vi "Create Folder.vi"(0 "Directory Path":path, 11 "error in (no error)":errorcluster) -> (4 "Dup Directory Path":path, 15 "error out":errorcluster)   [LabVIEW 2021, in "Path Functions.lvlib"]
uses:
  Path Functions.lvlib
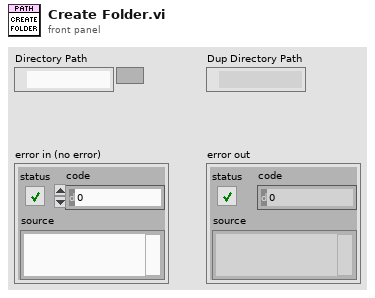
[diagram p1: front panel]
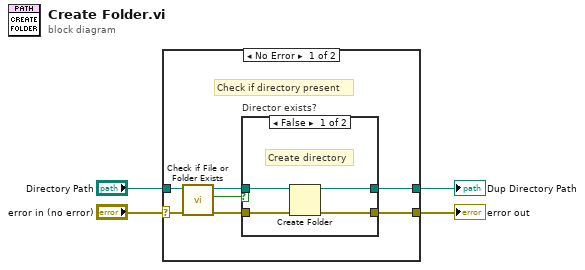
[diagram p0: block diagram]
diagram:
  n1 = case shown="No Error" "error in (no error)" {
    selector: "error in (no error)" -> [w11 w19]
    tunnel: "Directory Path" -> [w10 w18]
    tunnel: [w9 w19] -> w2
    tunnel: [w6 w18] -> w1
    frame No Error {
      # "Check if directory present"
      n2 = call <vilib>:"Check if File or Folder Exists.vi"("error in (no error)"=w11, "path"=w10) -> ("error out"=w8:errorcluster, "file or folder exists?"=w5:bool, "dup path"=w7:path)  [unwired: 7 in]
      n3 = case "Director exists?" shown="False" w5 {
        tunnel: w8 -> [w15 w17]
        tunnel: [w14 w17] -> w9
        tunnel: w7 -> [w13 w16]
        tunnel: [w12 w16] -> w6
        frame False {
          # "Create directory"
          n4 = Create Folder(path (use dialog)=w13, error in=w15) -> (created path=w12:path, error out=w14:errorcluster)  [unwired: 1 in, 1 out]
        }
        frame True {
        }
      }
    }
    frame Error {
    }
  }
  "error out" <- w2
  "Dup Directory Path" <- w1
